vi "Pre-Install Custom Action.vi"(10 "Variant":variant) -> (0 "error out":errorcluster)   [LabVIEW 2020]
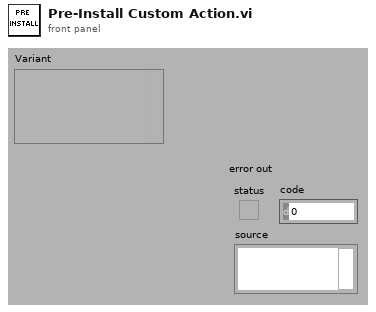
[diagram p1: front panel]
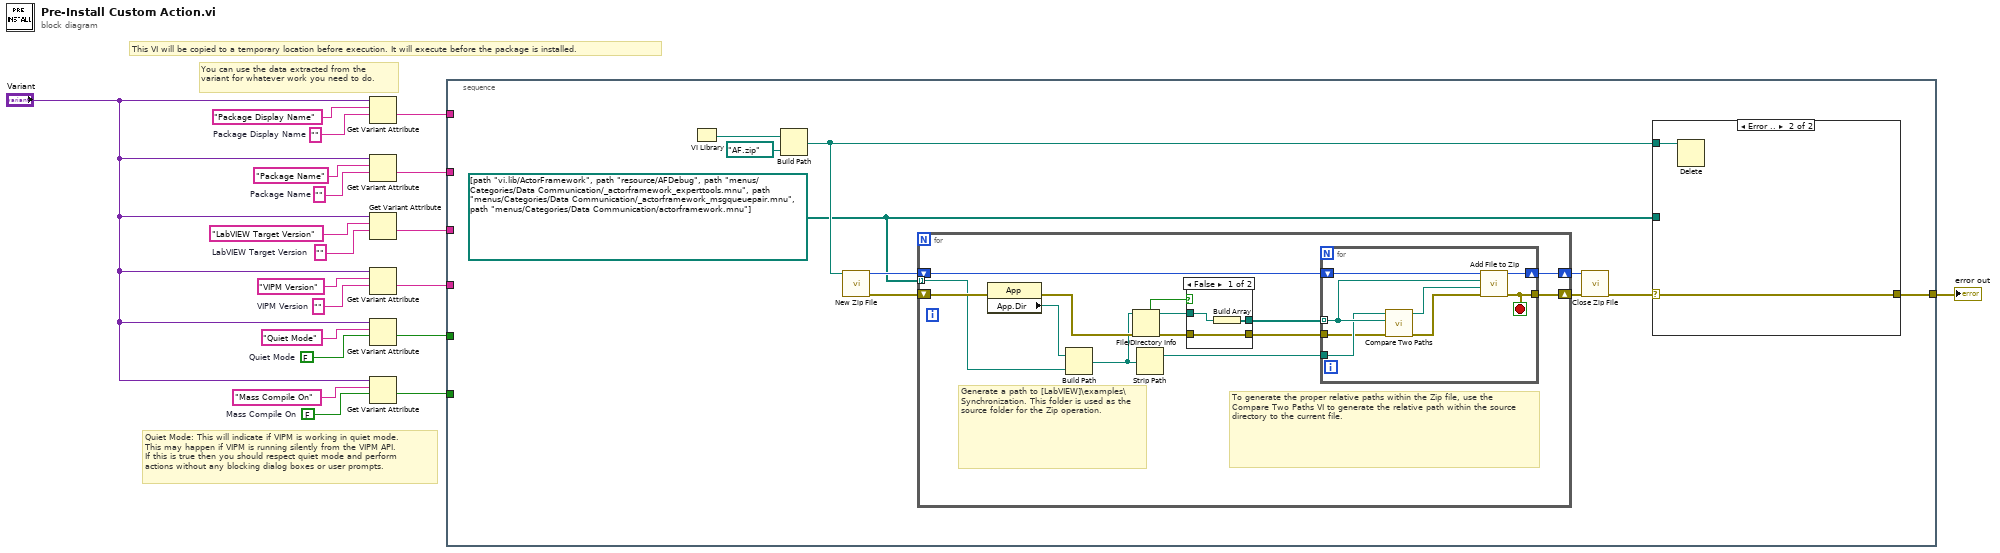
[diagram p0: block diagram]
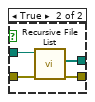
[diagram p2: hidden frame]
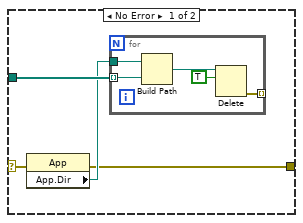
[diagram p3: hidden frame]
diagram:
  w2 = FALSE  # Mass Compile On
  w4 = ""  # Package Display Name
  w11 = FALSE  # Quiet Mode
  w14 = ""  # VIPM Version
  w16 = ""  # LabVIEW Target Version
  w18 = ""  # Package Name
  # "You can use the data extracted from the variant for whatever work you need to do."
  # "Quiet Mode: This will indicate if VIPM is working in quiet mode.\nThis may happen if VIPM is running silently from the VIPM API.\nIf this is true then you should respect quiet mode and perform\nactions without any blocking dialog boxes or user prompts."
  # "This VI will be copied to a temporary location before execution. It will execute before the package is installed."
  n1 = Get Variant Attribute(Variant="Variant", name="Package Display Name", default value (empty Variant)=w4) -> (value=w10:string)  [unwired: 1 in, 3 out]
  n2 = Get Variant Attribute(Variant="Variant", name="Package Name", default value (empty Variant)=w18) -> (value=w9:string)  [unwired: 1 in, 3 out]
  n3 = Get Variant Attribute(Variant="Variant", name="LabVIEW Target Version", default value (empty Variant)=w16) -> (value=w8:string)  [unwired: 1 in, 3 out]
  n4 = Get Variant Attribute(Variant="Variant", name="VIPM Version", default value (empty Variant)=w14) -> (value=w7:string)  [unwired: 1 in, 3 out]
  n5 = Get Variant Attribute(Variant="Variant", name="Quiet Mode", default value (empty Variant)=w11) -> (value=w6:bool)  [unwired: 1 in, 3 out]
  n6 = Get Variant Attribute(Variant="Variant", name="Mass Compile On", default value (empty Variant)=w2) -> (value=w5:bool)  [unwired: 1 in, 3 out]
  n7 = stacked-sequence {
    tunnel: w10 -> [_]
    tunnel: w9 -> [_]
    tunnel: w8 -> [_]
    tunnel: w7 -> [_]
    tunnel: w6 -> [_]
    tunnel: w5 -> [_]
    tunnel: [w30] -> w1
    frame #0 {
      w21 = path[] [path "vi.lib/ActorFramework", path "resource/AFDebug", path "menus/Categories/Data Communication/_actorframework_experttools.mnu", path "menus/Categories/Data Communication/_actorframework_msgqueuepair.mnu", path "menus/Categories/Data Communication/actorframework.mnu"]
      n8 = VI Library() -> (path=w23:path)
      n9 = Build Path(base path=w23, name or relative path=path "AF.zip") -> (appended path=w29:path)
      n10 = call <vilib>:"New Zip File.vi"("target"=w29) -> ("error out"=w25:errorcluster, "zip file out"=w24:i64)  [unwired: 2 in, 3 out]
      n11 = for {
        shift-right: [w43] -> w26
        shift-left: w25 -> [w44]
        tunnel: w21 -> [w42] mode=indexing
        shift-right: [w31] -> w27
        shift-left: w24 -> [w41]
        # "Generate a path to [LabVIEW]\\examples\\Synchronization. This folder is used as the source folder for the Zip operation."
        # "To generate the proper relative paths within the Zip file, use the Compare Two Paths VI to generate the relative path within the source directory to the current file."
        n12 = property class="App"(error in=w44) -> (error out=w40:errorcluster, "App.Dir"=w33:path)  [unwired: 1 in, 1 out]
        n13 = Build Path(base path=w33, name or relative path=w42) -> (appended path=w36:path)
        n14 = File/Directory Info(path=w36, error in=w40) -> (path out=w37:path, directory=w38:bool, error out=w35:errorcluster)  [unwired: 4 out]
        n15 = Strip Path(path=w36) -> (stripped path=w39:path)  [unwired: 1 out]
        n16 = case shown="False" w38 {
          tunnel: [w45 w51] -> w32
          tunnel: [w47 w50] -> w34
          tunnel: w35 -> [w47 w49]
          tunnel: w37 -> [w46 w48]
          frame False {
            n17 = Build Array(w46) -> (w45:path[])
          }
          frame True {
            n18 = call <vilib>:"Recursive File List.vi"("error in (no error)"=w49, "Folder Path"=w48) -> ("error out"=w50:errorcluster, "All Files in Dir"=w51:path[])  [unwired: 5 in, 3 out]
          }
        }
        n19 = for {
          tunnel: w32 -> [w56] mode=indexing
          tunnel: w34 -> [w53]
          tunnel: [w57] -> w43
          shift-right: [w58] -> w31
          shift-left: w41 -> [w59]
          tunnel: w39 -> [w55]
          stop <- w57 stop-if-true
          n20 = call <vilib>:"Compare Two Paths.vi"("error in (no error)"=w53, "Path 2"=w56, "Path 1"=w55) -> ("error out"=w52:errorcluster, "Relative Path from 1 to 2"=w54:path)  [unwired: 5 in, 2 out]
          n21 = call <vilib>:"Add File to Zip.vi"("error in (no error)"=w52, "destination path in zip"=w54, "source file path"=w56, "zip file in"=w59) -> ("error out"=w57:errorcluster, "zip file out"=w58:i64)  [unwired: 6 out]
        }
      }
      n22 = call <vilib>:"Close Zip File.vi"("error in (no error)"=w26, "zip file in"=w27) -> ("error out"=w28:errorcluster)  [unwired: 1 in, 4 out]
      n23 = case shown="Error .." w28 {
        selector: w28 -> [w63 w70]
        tunnel: [w60 w70] -> w30
        tunnel: w29 -> [_ w69]
        tunnel: w21 -> [w62 _]
        frame No Error {
          n24 = property class="App"(error in=w63) -> (error out=w60:errorcluster, "App.Dir"=w61:path)  [unwired: 1 in, 1 out]
          n25 = for {
            tunnel: w62 -> [w68] mode=indexing
            tunnel: w61 -> [w66]
            tunnel: [w65] -> _ mode=indexing
            n26 = Build Path(base path=w66, name or relative path=w68) -> (appended path=w67:path)
            n27 = Delete(path (use dialog)=w67, entire hierarchy (F)=TRUE) -> (error out=w65:errorcluster)  [unwired: 3 in, 2 out]
          }
        }
        frame Error {
          n28 = Delete(path (use dialog)=w69) -> ()  [unwired: 4 in, 3 out]
        }
      }
    }
  }
  "error out" <- w1
